vi "Table-UpdateDescriptionInd.vi"(8 "error in (no error)":errorcluster, 11 "ERP-SpecificationManager in":refnum<class "ERP-SpecificationManager.lvclass">) -> (0 "error out":errorcluster, 3 "ERP-SpecificationManager out":refnum<class "ERP-SpecificationManager.lvclass">)   [LabVIEW 2013, in "ERP-SpecificationManager.lvclass"]
uses:
  ERP-SpecificationManager.lvclass
  ERP-SpecificationManager.lvclass/ERP-SpecificationManager.ctl
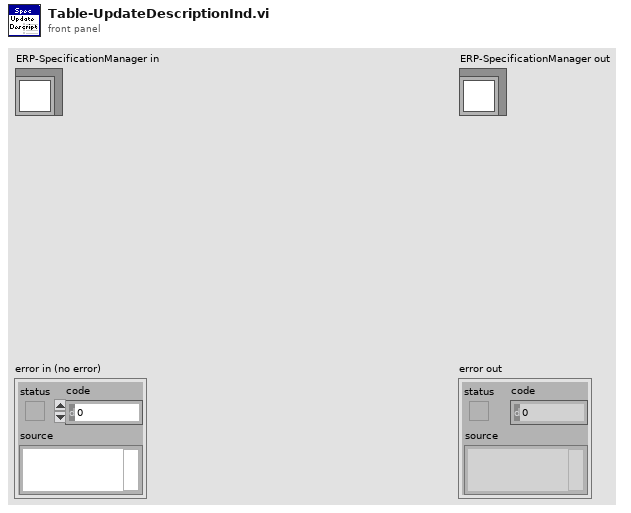
[diagram p1: front panel]
types:
  T1 = typedef "LVRowAndColumnTypeDef.ctl" = cluster{"Row":i32, "Column":i32}
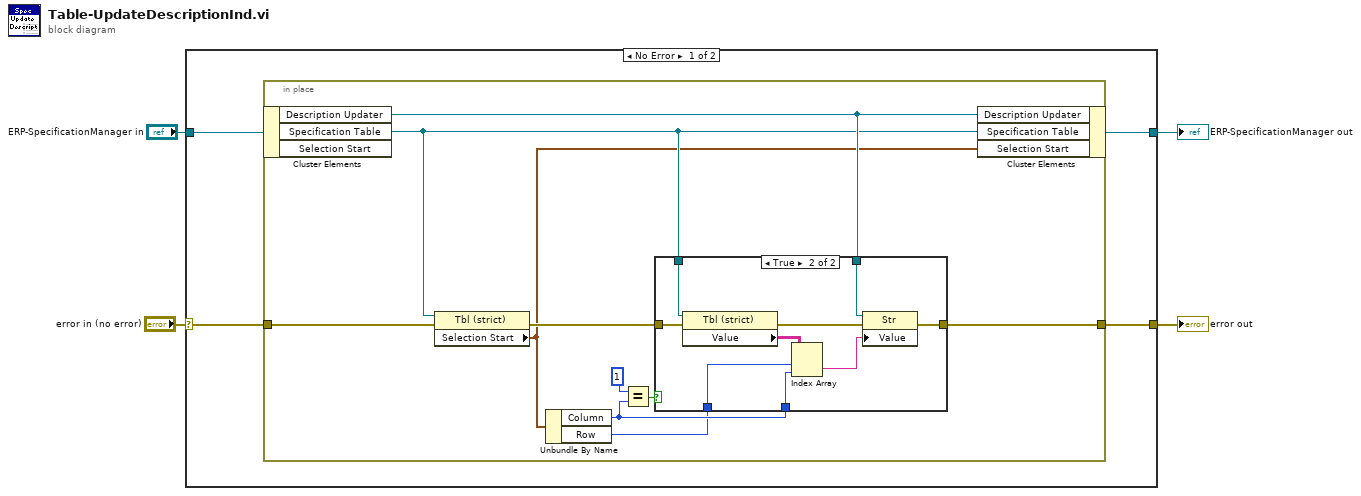
[diagram p0: block diagram]
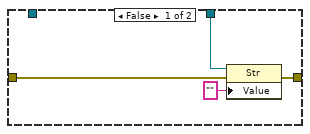
[diagram p2: hidden frame]
diagram:
  n1 = case shown="No Error" "error in (no error)" {
    selector: "error in (no error)" -> [w8 w33]
    tunnel: [w7 w33] -> w3
    tunnel: [w5 w32] -> w1
    tunnel: "ERP-SpecificationManager in" -> [w6 w32]
    frame No Error {
      n2 = in-place {
        in-place-border: w8 -> [w10]
        in-place-border: [w9] -> w7
        n3 = in-place-cluster #1(w6) -> ("Description Updater"=w13:refnum<vi>, "Specification Table"=w12:refnum<vi>)  [unwired: 1 out]
        n4 = property class="Tbl (strict)"(reference=w12, error in=w10) -> (error out=w15:errorcluster, "Selection Start"=w11:T1)  [unwired: 1 out]
        n5 = Unbundle By Name(w11) -> ("Column"=w18:i32, "Row"=w17:i32)
        n6 = Equal?(x=1, y=w18) -> (x = y?=w16:bool)
        n7 = case shown="True" w16 {
          tunnel: w12 -> [_ w31]
          tunnel: w15 -> [w22 w30]
          tunnel: w13 -> [w21 w28]
          tunnel: w17 -> [_ w26]
          tunnel: w18 -> [_ w25]
          tunnel: [w19 w23] -> w9
          frame False {
            n8 = property class="Str"(reference=w21, error in=w22, "Value"="") -> (error out=w19:errorcluster)  [unwired: 1 out]
          }
          frame True {
            n9 = property class="Tbl (strict)"(reference=w31, error in=w30) -> (error out=w27:errorcluster, "Value"=w29:string[][])  [unwired: 1 out]
            n10 = Index Array(array=w29, index (row)=w26, index (col)=w25) -> (element=w24:string)
            n11 = property class="Str"(reference=w28, error in=w27, "Value"=w24) -> (error out=w23:errorcluster)  [unwired: 1 out]
          }
        }
        n12 = in-place-cluster #1("Description Updater"=w13, "Specification Table"=w12, "Selection Start"=w11) -> (w5:refnum<class "ERP-SpecificationManager.lvclass">)
      }
    }
    frame Error {
    }
  }
  "error out" <- w3
  "ERP-SpecificationManager out" <- w1
